vi "SQL_Table_Unit_Test_Pressure_Insert.vi"(10 "时间标识":timestamp, 11 "液压子系统数据":T1) -> (3 "error out":errorcluster)   [LabVIEW 2014]
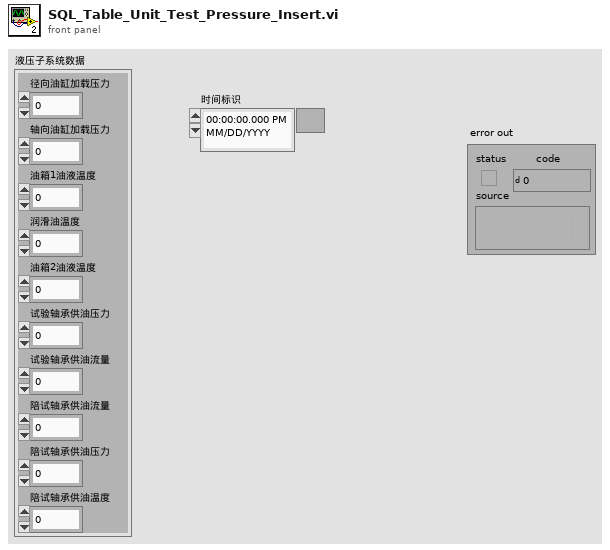
[diagram p1: front panel]
types:
  T1 = cluster{"径向油缸加载压力":u16, "轴向油缸加载压力":u16, "油箱1油液温度":u16, "润滑油温度":u16, "油箱2油液温度":u16, "试验轴承供油压力":u16, "试验轴承供油流量":u16, "陪试轴承供油流量":u16, "陪试轴承供油压力":u16, "陪试轴承供油温度":u16}
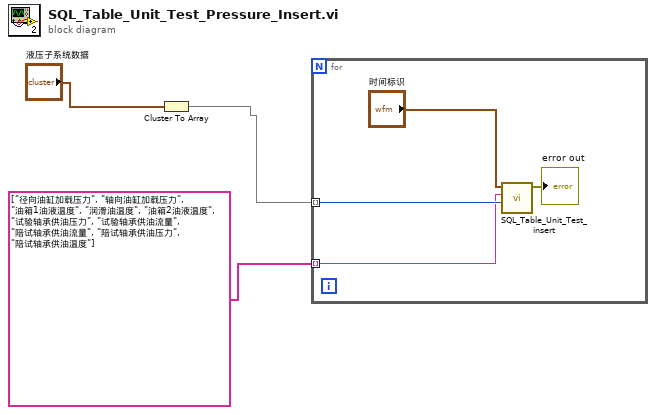
[diagram p0: block diagram]
diagram:
  n1 = Cluster To Array(cluster="液压子系统数据") -> (array=w1:u16[])
  n2 = for {
    tunnel: w1 -> [w6] mode=indexing
    tunnel: string[] ["径向油缸加载压力", "轴向油缸加载压力", "油箱1油液温度", "润滑油温度", "油箱2油液温度", "试验轴承供油压力", "试验轴承供油流量", "陪试轴承供油流量", "陪试轴承供油压力", "陪试轴承供油温度"] -> [w5] mode=indexing
    n3 = call "SQL_Table_Unit_Test_insert.vi"("数据数值"=w6, "数据名称"=w5, "时间标识"="时间标识") -> ("error out"=→"error out":errorcluster)  [unwired: 8 in]
  }
